vi "Relay Initialization.vi"   [LabVIEW 2015]
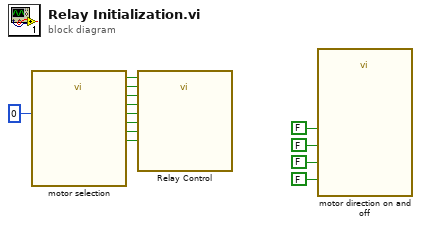
[diagram p0: block diagram]
diagram:
  n1 = call "motor selection.vi"("index 2"=0) -> ("[0]"=w13:bool, "[1]"=w12:bool, "[2]"=w11:bool, "[3]"=w10:bool, "[4]"=w9:bool, "[5]"=w8:bool, "[6]"=w7:bool, "[7]"=w6:bool)  [unwired: 19 in]
  n2 = call "Relay Control.vi"("State 8"=w13, "State 9"=w12, "State 10"=w11, "State 11"=w10, "State 12"=w9, "State 13"=w8, "State 14"=w7, "State 15"=w6) -> ()  [unwired: 20 in]
  n3 = call "motor direction on and off.vi"("State 3"=FALSE, "State 2"=FALSE, "State 1"=FALSE, "State 0"=FALSE) -> ()  [unwired: 8 in]
